vi "testVI.vi"() -> ()   [LabVIEW 2013]
uses:
  Shared/GUI_Template/GUI_master/tcp new data cluster.ctl
panel:
  in  "stop":bool=TRUE
  in  "Trigger.Low Level::1":dbl=-1.0 min=0.0 max=10.0
  out "GUIdevice 1":string="StagingPXISlow"
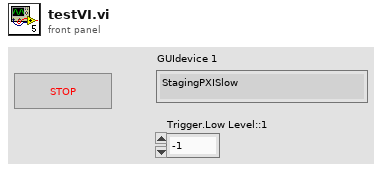
[diagram p1: front panel]
types:
  T1 = typedef "tcp new data cluster.ctl" = cluster{"EventEnum":enum16{"new data", "connection status update"}, "Device name":string}
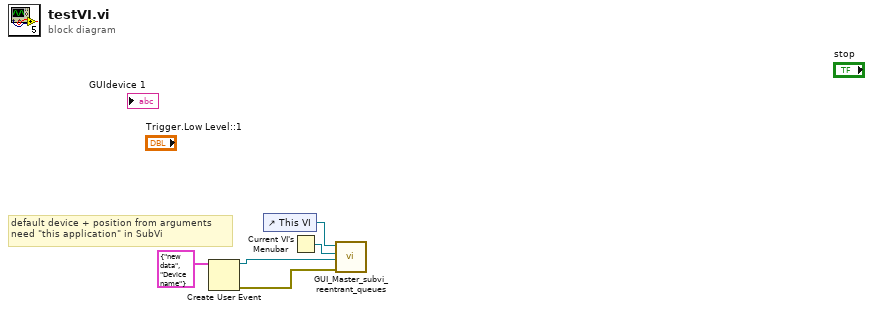
[diagram p0: block diagram]
diagram:
  # "default device + position from arguments\nneed \"this application\" in SubVi"
  n1 = Create User Event(user event datatype=T1 {"EventEnum"=enum."new data", "Device name"="Device name"} ("New Event")) -> (user event=w1:refnum<user-event>, error out=w2:errorcluster)  [unwired: 1 in]
  n2 = control-ref of="This VI"() -> (w5:refnum<vi>)
  n3 = Current VI's Menubar() -> (w4:refnum<k9>)
  n4 = call "GUI_Master_subvi_reentrant_queues.vi"("error in (no error)"=w2, "tcp data event"=w1, "Caller menu reference"=w4, "Caller VI ref"=w5) -> ()  [unwired: 7 in, 1 out]
